vi "RyanRemove.vi"(10 "Boolean":bool, 11 "IN":dbl[](array[numeric])) -> (3 "OUT":dbl[](array[numeric]))   [LabVIEW 2016]
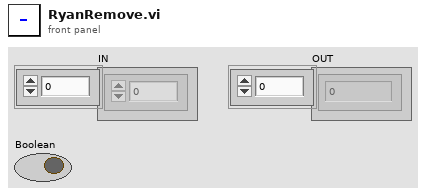
[diagram p1: front panel]
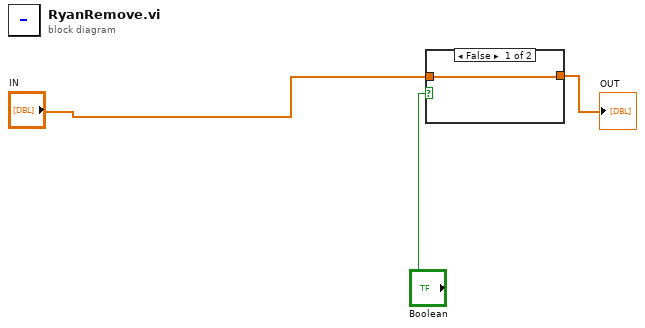
[diagram p0: block diagram]
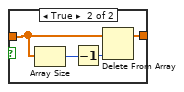
[diagram p2: hidden frame]
diagram:
  n1 = case shown="False" "Boolean" {
    tunnel: "IN" -> [w4 w8]
    tunnel: [w4 w7] -> w2
    frame False {
    }
    frame True {
      n2 = Array Size(array=w8) -> (size(s)=w6:i32)
      n3 = Decrement(x=w6) -> (x-1=w5:i32)
      n4 = Delete From Array(array=w8, index=w5) -> (array with subset deleted=w7:dbl[])  [unwired: 1 in, 1 out]
    }
  }
  "OUT" <- w2
